vi "Validate & Instantiate Functions.vi"(0 "Functions in":T1[](array[typedef]), 1 "function manager":refnum<class "function manager.lvclass">, 11 "error in (no error)":errorcluster) -> (4 "Function":T1[](array[typedef]), 6 "Function [obj]":refnum<class "functionbase.lvclass">[](array[class]), 8 "Comiplation message":T2[](array[typedef]), 15 "error out":errorcluster)   [LabVIEW 2016, in "scripts manager.lvclass"]
uses:
  scripts manager.lvclass
  common/Line Details.ctl
  functions/function utils/function manager.lvclass
  common/Validate_message.ctl
  functions/functionsbase/functionbase.lvclass
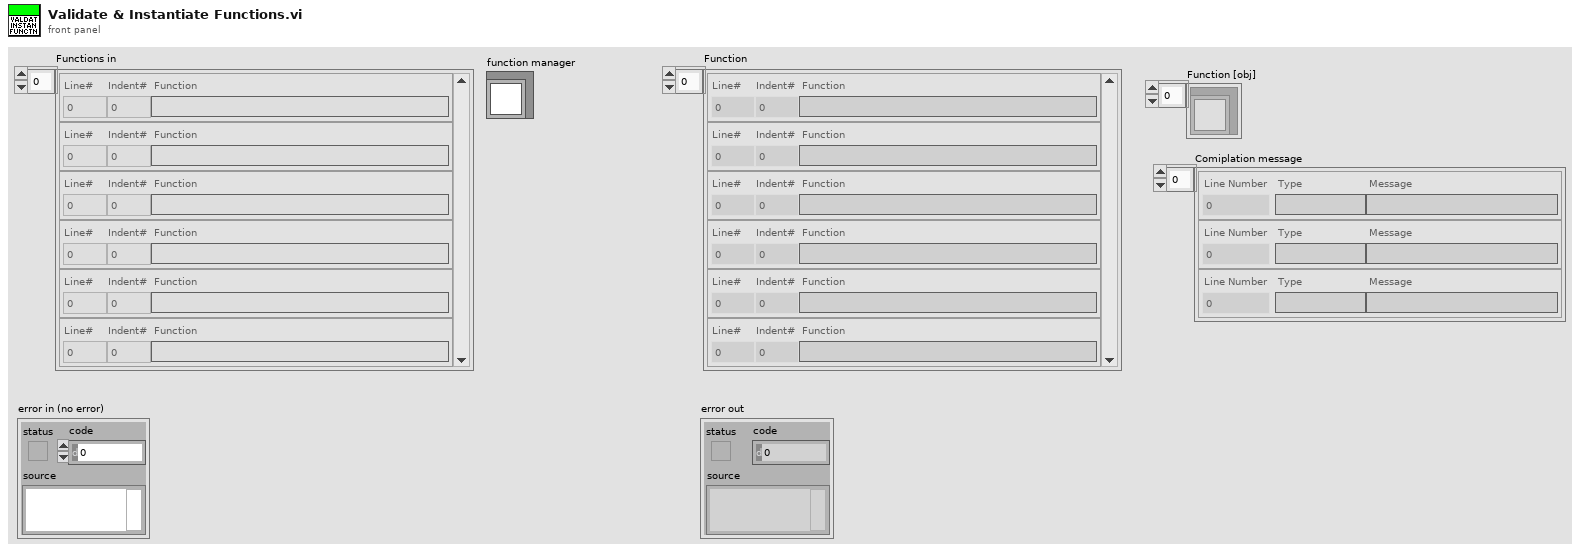
[diagram p1: front panel]
types:
  T1 = typedef "Line Details.ctl" = cluster{"Line#":i64, "Indent#":i64, "Function":string}
  T2 = typedef "Validate_message.ctl" = cluster{"Line Number":i64, "Type":string, "Message":string}
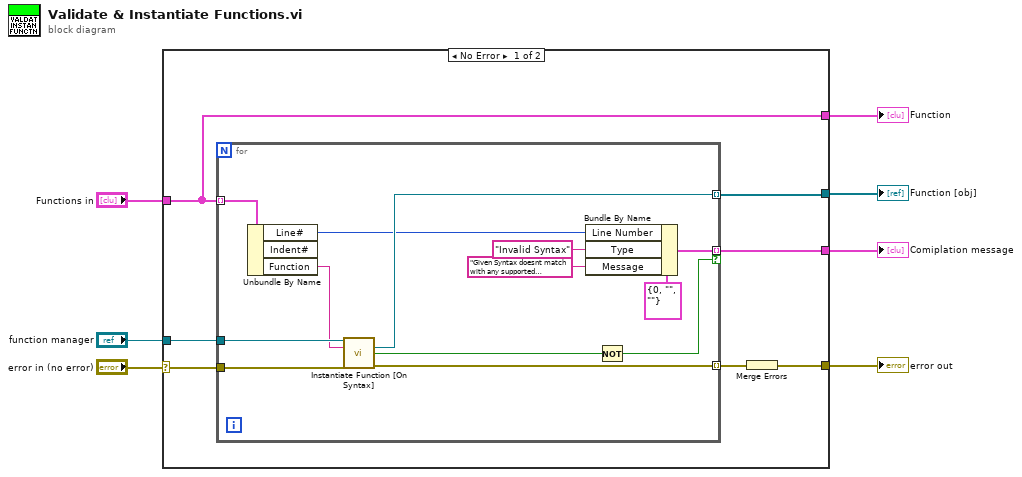
[diagram p0: block diagram]
diagram:
  n1 = case shown="No Error" "error in (no error)" {
    selector: "error in (no error)" -> [w13 w28]
    tunnel: [w11 w28] -> w6
    tunnel: "Functions in" -> [w8 _]
    tunnel: "function manager" -> [w14 _]
    tunnel: [w10 _] -> w3
    tunnel: [w9 _] -> w2
    tunnel: [w8 _] -> w1
    frame No Error {
      n2 = for {
        tunnel: w8 -> [w27] mode=indexing
        tunnel: w14 -> [w26]
        tunnel: w13 -> [w25]
        tunnel: [w23] -> w12 mode=indexing
        tunnel: [w22] -> w9 mode=indexing
        tunnel: [w20] -> w10 mode=indexing if=w18
        n3 = Unbundle By Name(w27) -> ("Line#"=w17:i64, "Function"=w24:string)  [unwired: 1 out]
        n4 = call "Instantiate Function [On Syntax].vi"("function manager in"=w26, "Function String"=w24, "error in (no error)"=w25) -> ("function obj"=w22:refnum<class "functionbase.lvclass">, "Valid Syntax?"=w19:bool, "error out"=w23:errorcluster)  [unwired: 9 in, 1 out]
        n5 = Bundle By Name(cluster=T2 {"Line Number"=0, "Type"="", "Message"=""} ("Message"), "Line Number"=w17, "Type"="Invalid Syntax", "Message"="Given Syntax doesnt match with any supported functions") -> (w20:T2)
        n6 = Not(x=w19) -> (.not. x?=w18:bool)
      }
      n7 = Merge Errors(w12) -> (w11:errorcluster)
    }
    frame Error {
    }
  }
  "error out" <- w6
  "Comiplation message" <- w3
  "Function [obj]" <- w2
  "Function" <- w1
